vi "Close.vi"(8 "error in (no error)":errorcluster, 11 "SGDV FPGA Target in":refnum<class "SGDV FPGA Target.lvclass">) -> (0 "error out":errorcluster, 3 "SGDV FPGA Target out":refnum<class "SGDV FPGA Target.lvclass">)   [LabVIEW 2013, in "SGDV_Ctrl_v13_lib.lvlib" / "SGDV FPGA Target.lvclass"]
uses:
  SGDV FPGA Target.lvclass
  SGDV FPGA Target.lvclass/SGDV FPGA Target.ctl
  SGDV_Ctrl_v13_lib.lvlib
  SGDV_Ctrl_Class/SGDV Motor.lvclass
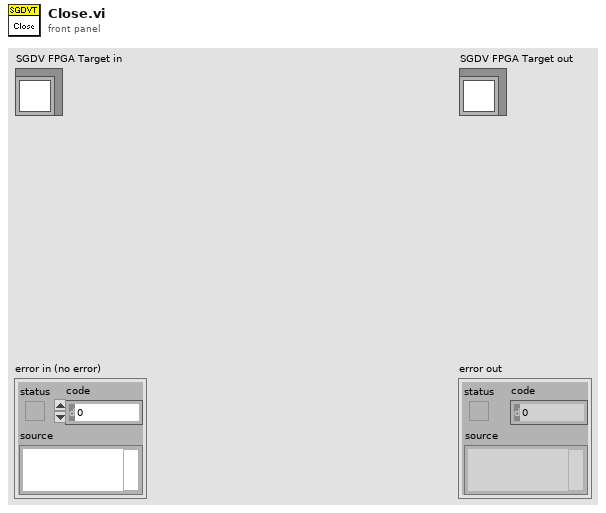
[diagram p1: front panel]
types:
  T1 = typedef "Generic FPGA Reference.ctl" = refnum<k20>
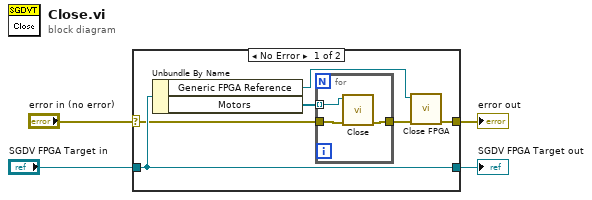
[diagram p0: block diagram]
diagram:
  n1 = case shown="No Error" "error in (no error)" {
    selector: "error in (no error)" -> [w8 w15]
    tunnel: [w5 w15] -> w3
    tunnel: [w10 w14] -> w1
    tunnel: "SGDV FPGA Target in" -> [w10 w14]
    frame No Error {
      n2 = Unbundle By Name(w10) -> ("Generic FPGA Reference"=w7:T1, "Motors"=w9:refnum<class "SGDV Motor.lvclass">[])
      n3 = for {
        tunnel: w9 -> [w13] mode=indexing
        tunnel: w8 -> [w12]
        tunnel: [w11] -> w6
        n4 = call "Close.vi"("error in (no error)"=w12, "SGDV_Ctrl_Class in"=w13) -> ("error out"=w11:errorcluster)  [unwired: 8 in, 1 out]
      }
      n5 = call "Close FPGA.vi"("error in (no error)"=w6, "Generic FPGA Reference"=w7) -> ("error out"=w5:errorcluster)  [unwired: 9 in]
    }
    frame Error {
    }
  }
  "error out" <- w3
  "SGDV FPGA Target out" <- w1
